vi "ErrorToDB.vi"(8 "Error":bool=TRUE, 9 "Folder":string, 10 "Command":string, 11 "Error Message":string) -> (2 "LogData":string)   [LabVIEW 2012]
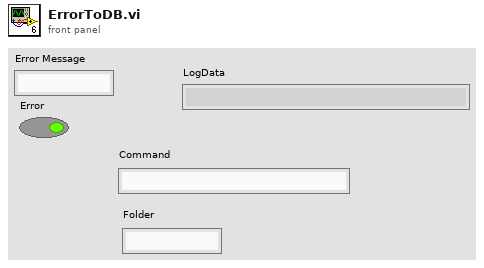
[diagram p1: front panel]
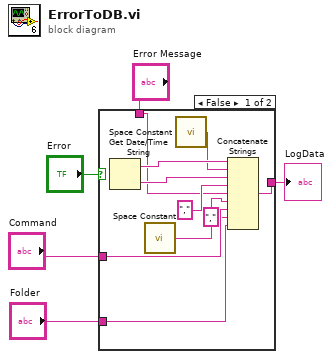
[diagram p0: block diagram]
diagram:
  n1 = case shown="False" "Error" {
    tunnel: [w11 w16] -> w3
    tunnel: "Error Message" -> [w10 w16]
    tunnel: "Command" -> [w8 _]
    tunnel: "Folder" -> [w6 _]
    frame False {
      n2 = Get Date/Time String() -> (date string=w13:string, time string=w14:string)  [unwired: 3 in]
      n3 = call <vilib>:"Space Constant.vi"() -> ("String"=w9:string)
      n4 = call <vilib>:"Space Constant.vi"() -> ("String"=w12:string)
      n5 = Concatenate Strings(w13, w12, w14, "," ("string"), w10, w9, w8, "," ("string"), w6) -> (w11:string)
    }
    frame True {
    }
  }
  "LogData" <- w3
